vi "Prepare Two Step Build.vi"(8 "error in (no error)":errorcluster, 11 "NI_AB_API_Build in":refnum<class "NI_AB_API_Build.lvclass">) -> (0 "error out":errorcluster, 2 "Build Context":refnum<vi>, 3 "NI_AB_API_Build out":refnum<class "NI_AB_API_Build.lvclass">)   [LabVIEW 2020, in "NI_AB_API_Build.lvclass"]
uses:
  <vilib>/AppBuilder/AB_API/Build/NI_AB_API_Build.lvclass
  <vilib>/AppBuilder/AB_API/Build/NI_AB_API_Build.lvclass/NI_AB_API_Build.ctl
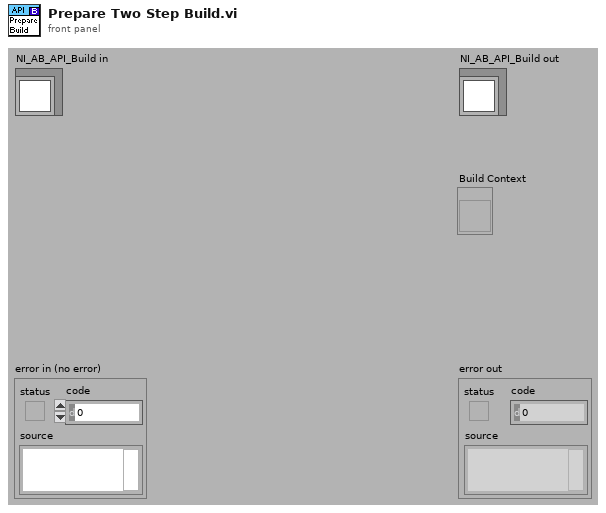
[diagram p1: front panel]
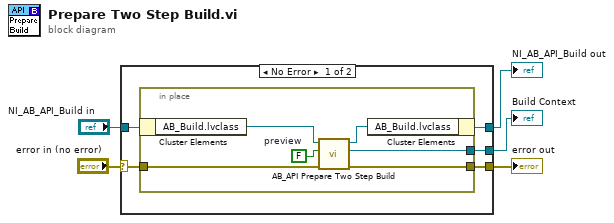
[diagram p0: block diagram]
diagram:
  n1 = case shown="No Error" "error in (no error)" {
    selector: "error in (no error)" -> [w9 w18]
    tunnel: [w8 w18] -> w4
    tunnel: [w6 w17] -> w2
    tunnel: "NI_AB_API_Build in" -> [w7 w17]
    tunnel: [w10 _] -> w1
    frame No Error {
      n2 = in-place {
        in-place-border: [w16] -> w10
        in-place-border: w9 -> [w15]
        in-place-border: [w14] -> w8
        w13 = FALSE  # preview
        n3 = in-place-cluster #1(w7) -> ("AB_Build.lvclass"=w12:refnum<class "AB_Build.lvclass">)
        n4 = call <vilib>:"AB_API Prepare Two Step Build.vi"("error in (no error)"=w15, "preview"=w13, "Build in"=w12) -> ("error out"=w14:errorcluster, "Build Context"=w16:refnum<vi>, "Class out"=w11:refnum<class "AB_Build.lvclass">)  [unwired: 6 in]
        n5 = in-place-cluster #1("AB_Build.lvclass"=w11) -> (w6:refnum<class "NI_AB_API_Build.lvclass">)
      }
    }
    frame Error {
    }
  }
  "error out" <- w4
  "NI_AB_API_Build out" <- w2
  "Build Context" <- w1
